vi "Decompose LabVIEW Object - Child - Library Version Value.vi"() -> ()   [LabVIEW 2017, in "Composition.Tests.lvlib"]
uses:
  Composition.Tests.lvlib
  Classes/Child/Child.lvclass
  Composition/Composition.lvlib
  <vilib>/addons/_JKI Toolkits/Caraya/classes/Assert/Assert.lvclass
  <vilib>/addons/_JKI Toolkits/Caraya/classes/Test/Test.lvclass
panel:
  out "error out":errorcluster
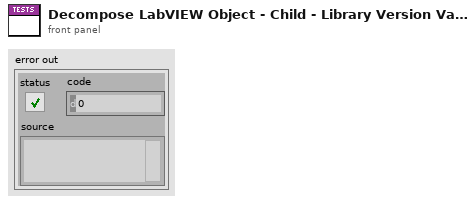
[diagram p1: front panel]
types:
  T1 = cluster{"Major":u16, "Minor":u16, "Fix":u16, "Build":u16}[]
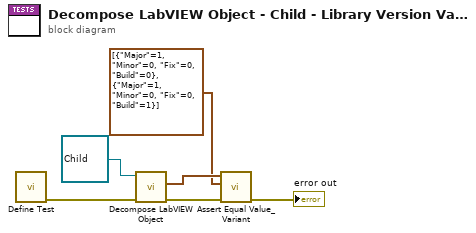
[diagram p0: block diagram]
diagram:
  n1 = call <vilib>:"Define Test.vi"() -> ("error out"=w1:errorcluster)  [unwired: 11 in]
  n2 = call "Decompose LabVIEW Object.vi"("error in (no error)"=w1, "LabVIEW Object"=refnum<class "Child.lvclass"> refnum ("Reflection.Tests.lvlib:Child.lvclass")) -> ("error out"=w5:errorcluster, "Library Versions"=w3:T1)  [unwired: 6 in, 2 out]
  n3 = call <vilib>:"Assert Equal Value_Variant.vi"("error in (no error)"=w5, "Y"=T1 [{"Major"=1, "Minor"=0, "Fix"=0, "Build"=0}, {"Major"=1, "Minor"=0, "Fix"=0, "Build"=1}] ("Library Versions"), "X"=w3) -> ("error out"=→"error out":errorcluster)  [unwired: 8 in]
